vi "Set Build Types.vi"(10 "Build Types":T1[](array[typedef]), 11 "CD Build Tools in":refnum<class "Project Build Tools.lvclass">) -> (3 "CD Build Tools out":refnum<class "Project Build Tools.lvclass">)   [LabVIEW 2019, in "Project Build Tools.lvclass"]
uses:
  Project Build Tools.lvclass
  TypeDefs/Configure Build Types.ctl
  Project Build Tools.lvclass/Project Build Tools.ctl
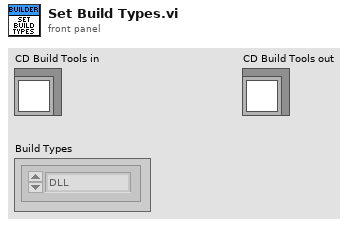
[diagram p1: front panel]
types:
  T1 = typedef "Project Build Tools.lvclass/Configure Build Types.ctl" = enum16{"DLL", "Packed Library", "Installer", "Source Distribution", "EXE"}
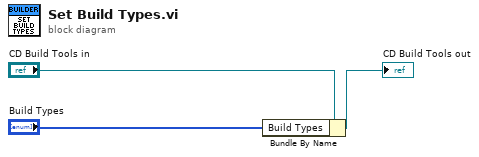
[diagram p0: block diagram]
diagram:
  n1 = Bundle By Name(cluster="CD Build Tools in", "Build Types"="Build Types") -> (→"CD Build Tools out":refnum<class "Project Build Tools.lvclass">)
